vi "Write Element of Array - String.vi"(8 "error in (no error)":errorcluster, 9 "String":string, 10 "index":i32, 11 "TAS_Message in":refnum<class "TAS_Message.lvclass">) -> (0 "error out":errorcluster, 3 "TAS_Message out":refnum<class "TAS_Message.lvclass">)   [LabVIEW 2012, in "TAS_Message.lvclass"]
uses:
  TAS_Message.lvclass
  TAS_Message.lvclass/TAS_Message.ctl
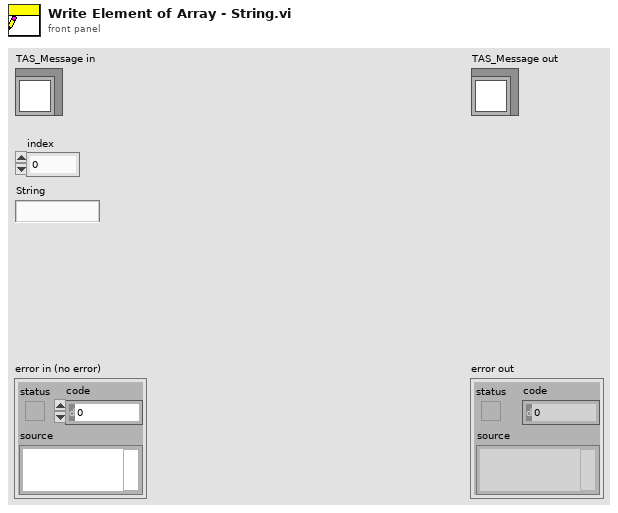
[diagram p1: front panel]
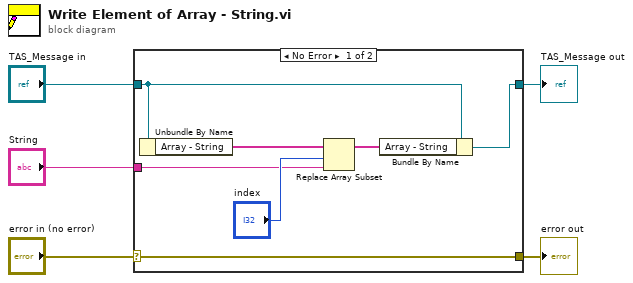
[diagram p0: block diagram]
diagram:
  n1 = case shown="No Error" "error in (no error)" {
    selector: "error in (no error)" -> [w12 w13]
    tunnel: [w12 w13] -> w4
    tunnel: [w11 w14] -> w2
    tunnel: "TAS_Message in" -> [w10 w14]
    tunnel: "String" -> [w6 _]
    frame No Error {
      n2 = Unbundle By Name(w10) -> ("Array - String"=w9:string[])
      n3 = Replace Array Subset(array=w9, new element=w6, index="index") -> (w8:string[])
      n4 = Bundle By Name(cluster=w10, "Array - String"=w8) -> (w11:refnum<class "TAS_Message.lvclass">)
    }
    frame Error {
    }
  }
  "error out" <- w4
  "TAS_Message out" <- w2
